vi "Untitled 15 (SubVI).vi"(9 "output bit stream":i8[](array[numeric]), 10 "Размер окна с паузами":i32, 11 "Кол-во копий":i32) -> (3 "Array":i8[][](array[numeric]))   [LabVIEW 2017]
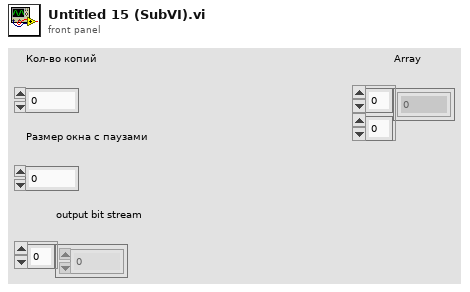
[diagram p1: front panel]
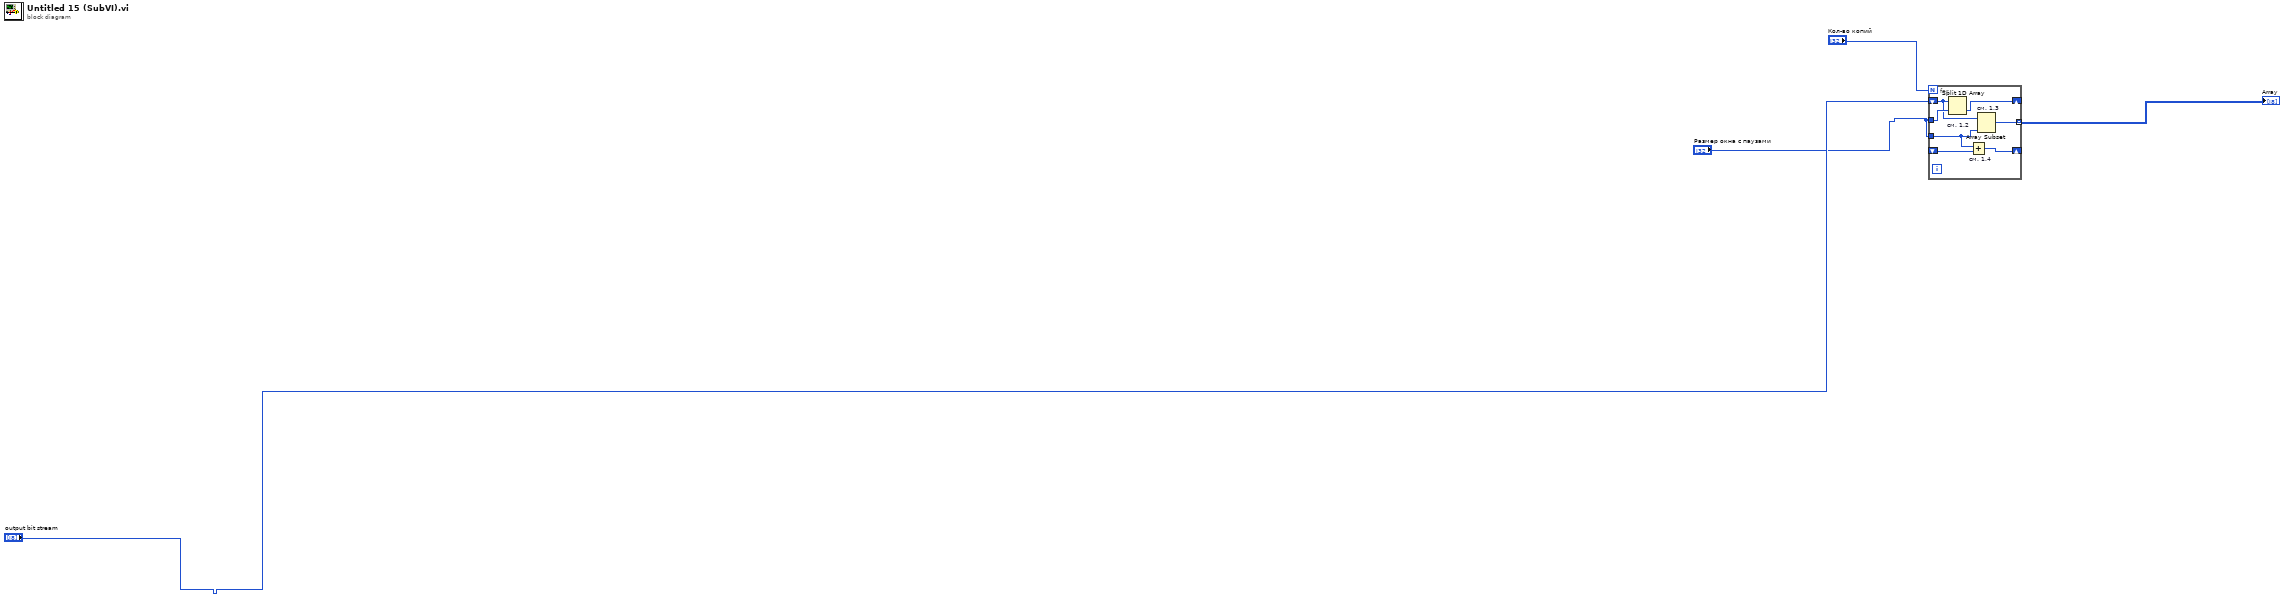
[diagram p0: block diagram]
diagram:
  n1 = for {
    N: "Кол-во копий" -> [_]
    shift-right: [w11] -> _
    shift-left: "output bit stream" -> [w9]
    tunnel: "Размер окна с паузами" -> [w10]
    shift-right: [w7] -> _
    shift-left: _ -> [w6]
    tunnel: "Размер окна с паузами" -> [w8]
    tunnel: [w5] -> w1 mode=indexing
    n2 = Split 1D Array "см. 1.2"(array=w9, index=w10) -> (second subarray=w11:i8[])  [unwired: 1 out]
    n3 = Add "см. 1.4"(x=w8, y=w6) -> (x+y=w7:i32)
    n4 = Array Subset "см. 1.3"(array=w9, length=w8) -> (w5:i8[])  [unwired: 1 in]
  }
  "Array" <- w1
